vi "Initialize Hardware References.vi"(8 "error in (no error)":errorcluster, 11 "Hardware Resources in":T1) -> (0 "error out":errorcluster, 3 "Hardware Resources out":T1)   [LabVIEW 2021, in "IMU Acquisition.lvlib"]
doc: "Initialize the hardware references."
uses:
  IMU Acquisition.lvlib
  Hardware Configuration.ctl
  Signal Type.ctl
  <vilib>/Instr/_visa.llb/VISA Configure Serial Port (Instr).vi
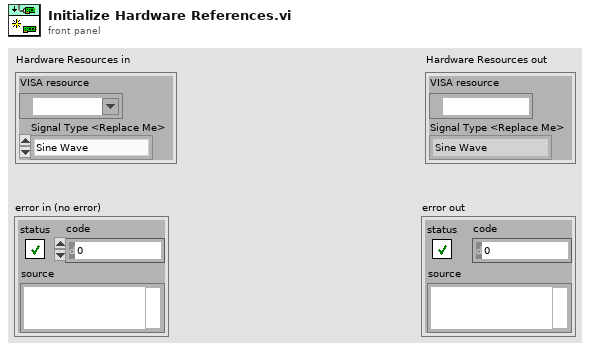
[diagram p1: front panel]
types:
  T1 = typedef "IMU Acquisition.lvlib/Hardware Configuration.ctl" = cluster{"VISA resource":refnum<visa-resource-name>, "Signal Type <Replace Me>":T2}
  T2 = typedef "IMU Acquisition.lvlib/Signal Type.ctl" = enum16{"Sine Wave", "Square with Noise"}
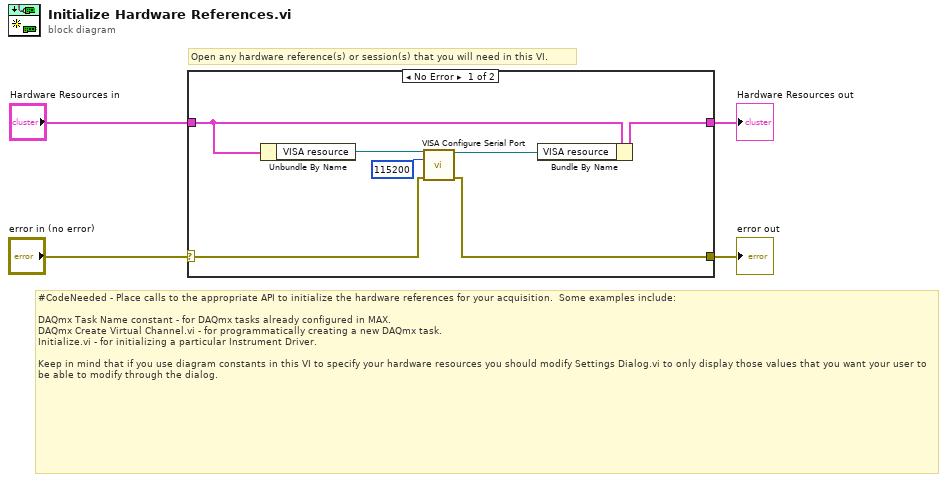
[diagram p0: block diagram]
diagram:
  # "Open any hardware reference(s) or session(s) that you will need in this VI."
  # "#CodeNeeded - Place calls to the appropriate API to initialize the hardware references for your acquisition.  Some examples include:\n\nDAQmx Task Name constant - for DAQmx tasks already configured in MAX.\nDAQmx Create Virtual Channel.vi - for programmatically creating a new DAQmx task.\nInitialize.vi - for initializing a particular Instrument Driver.\n\nKeep in mind that if you use diagram constants in this VI to specify your hardware resources you should modify Settings Dialog.vi to only display those values that you want your user to be able to modify through the dialog."
  n1 = case shown="No Error" "error in (no error)" {
    selector: "error in (no error)" -> [w6 w12]
    tunnel: [w5 w12] -> w3
    tunnel: "Hardware Resources in" -> [w10 w13]
    tunnel: [w11 w13] -> w1
    frame No Error {
      n2 = Unbundle By Name(w10) -> ("VISA resource"=w9:refnum<visa-resource-name>)
      n3 = call-poly "VISA Configure Serial Port"("VISA resource name"=w9, "baud rate (9600)"=u32 115200, "error in (no error)"=w6) -> ("VISA resource name out"=w8:refnum<visa-resource-name>, "error out"=w5:errorcluster)  [unwired: 11 in]
      n4 = Bundle By Name(cluster=w10, "VISA resource"=w8) -> (w11:T1)
    }
    frame Error {
    }
  }
  "Hardware Resources out" <- w1
  "error out" <- w3
